vi "Multiply Force.vi"(10 "force in":dbl, 11 "Bottle Opener in":refnum<class "Bottle Opener.lvclass">) -> (2 "force out":dbl)   [LabVIEW 2023, in "Bottle Opener.lvclass"]
uses:
  Bottle Opener.lvclass
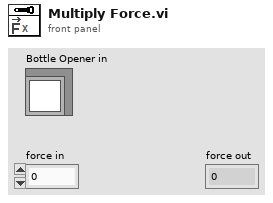
[diagram p1: front panel]
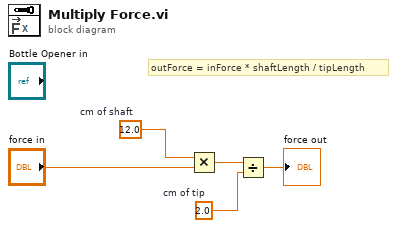
[diagram p0: block diagram]
diagram:
  w1 = 12.0  # cm of shaft
  w2 = 2.0  # cm of tip
  # "outForce = inForce * shaftLength / tipLength"
  n1 = Multiply(x=w1, y="force in") -> (x*y=w4:dbl)
  n2 = Divide(x=w4, y=w2) -> (x/y=→"force out":dbl)
